vi "APC_9049_CycleAvgSignals.vi"() -> (1 "CRIo9049_CycleAvgSignals":string[](array[string])=["TimeStamp9049_ms", "TimeStamp9056echo_ms", "InjectionState_b", "InjEnable_b", "MainEnable_b", "MainDuration_ms", "MainSOI_CADBTDC", "SparkEnable_b", "SparkTiming_CADBTDC", "EngineSpeed_rpm", "WF-PT-012avg_bar", "WF-PT-005avg_bar", "IMEPg1_bar", "IMEPg2_bar", "IMEPg3_bar", "IMEPg4_bar", "IMEPg5_bar", "IMEPg6_bar", "IMEPn1_bar", "IMEPn2_bar", "IMEPn3_bar", "IMEPn4_bar", "IMEPn5_bar", "IMEPn6_bar", "PMEP1_bar", "PMEP2_bar", "PMEP3_bar", "PMEP4_bar", "PMEP5_bar", "PMEP6_bar", "MaxPcyl1_bar", "MaxPcyl2_bar", "MaxPcyl3_bar", "MaxPcyl4_bar", "MaxPcyl5_bar", "MaxPcyl6_bar", "IMEPstd1_bar", "IMEPstd2_bar", "IMEPstd3_bar", "IMEPstd4_bar", "IMEPstd5_bar", "IMEPstd6_bar", "MAPO1_bar", "MAPO2_bar", "MAPO3_bar", "MAPO4_bar", "MAPO5_bar", "MAPO6_bar", "RI1", "RI2", "RI3", "RI4", "RI5", "RI6", "maxQ1_J", "maxQ2_J", "maxQ3_J", "maxQ4_J", "maxQ5_J", "maxQ6_J", "CA03_1_CADATDC", "CA03_2_CADATDC", "CA03_3_CADATDC", "CA03_4_CADATDC", "CA03_5_CADATDC", "CA03_6_CADATDC", "CA10_1_CADATDC", "CA10_2_CADATDC", "CA10_3_CADATDC", "CA10_4_CADATDC", "CA10_5_CADATDC", "CA10_6_CADATDC", "CA50_1_CADATDC", "CA50_2_CADATDC", "CA50_3_CADATDC", "CA50_4_CADATDC", "CA50_5_CADATDC", "CA50_6_CADATDC", "CA90_1_CADATDC", "CA90_2_CADATDC", "CA90_3_CADATDC", "CA90_4_CADATDC", "CA90_5_CADATDC", "CA90_6_CADATDC", "CA97_1_CADATDC", "CA97_2_CADATDC", "CA97_3_CADATDC", "CA97_4_CADATDC", "CA97_5_CADATDC", "CA97_6_CADATDC", "CA10CA90_1_CAD", "CA10CA90_2_CAD", "CA10CA90_3_CAD", "CA10CA90_4_CAD", "CA10CA90_5_CAD", "CA10CA90_6_CAD", "maxdpdcad1_barCAD", "maxdpdcad2_barCAD", "maxdpdcad3_barCAD", "maxdpdcad4_barCAD", "maxdpdcad5_barCAD", "maxdpdcad6_barCAD", "kappa_comp1_r", "kappa_comp2_r", "kappa_comp3_r", "kappa_comp4_r", "kappa_comp5_r", "kappa_comp6_r", "kappa_exp1_r", "kappa_exp2_r", "kappa_exp3_r", "kappa_exp4_r", "kappa_exp5_r", "kappa_exp6_r", "CylPresWarnings_u64", "CylPresErrors_u64"])   [LabVIEW 2020]
panel:
  in  "CycleRaster":string[](array[string])=["WF-PT-012avg_bar", "WF-PT-005avg_bar", "PrechamberPeakPdiff_bar", "IMEPg1_bar", "IMEPg2_bar", "IMEPg3_bar", "IMEPg4_bar", "IMEPg5_bar", "IMEPg6_bar", "IMEPn1_bar", "IMEPn2_bar", "IMEPn3_bar", "IMEPn4_bar", "IMEPn5_bar", "IMEPn6_bar", "PMEP1_bar", "PMEP2_bar", "PMEP3_bar", "PMEP4_bar", "PMEP5_bar", "PMEP6_bar", "MaxPcyl1_bar", "MaxPcyl2_bar", "MaxPcyl3_bar", "MaxPcyl4_bar", "MaxPcyl5_bar", "MaxPcyl6_bar", "IMEPstd1_bar", "IMEPstd2_bar", "IMEPstd3_bar", "IMEPstd4_bar", "IMEPstd5_bar", "IMEPstd6_bar", "MAPO1_bar", "MAPO2_bar", "MAPO3_bar", "MAPO4_bar", "MAPO5_bar", "MAPO6_bar", "RI1", "RI2", "RI3", "RI4", "RI5", "RI6", "maxQ1_J", "maxQ2_J", "maxQ3_J", "maxQ4_J", "maxQ5_J", "maxQ6_J", "CA03_1_CADATDC", "CA03_2_CADATDC", "CA03_3_CADATDC", "CA03_4_CADATDC", "CA03_5_CADATDC", "CA03_6_CADATDC", "CA10_1_CADATDC", "CA10_2_CADATDC", "CA10_3_CADATDC", "CA10_4_CADATDC", "CA10_5_CADATDC", "CA10_6_CADATDC", "CA50_1_CADATDC", "CA50_2_CADATDC", "CA50_3_CADATDC", "CA50_4_CADATDC", "CA50_5_CADATDC", "CA50_6_CADATDC", "CA90_1_CADATDC", "CA90_2_CADATDC", "CA90_3_CADATDC", "CA90_4_CADATDC", "CA90_5_CADATDC", "CA90_6_CADATDC", "CA97_1_CADATDC", "CA97_2_CADATDC", "CA97_3_CADATDC", "CA97_4_CADATDC", "CA97_5_CADATDC", "CA97_6_CADATDC", "CA10CA90_1_CAD", "CA10CA90_2_CAD", "CA10CA90_3_CAD", "CA10CA90_4_CAD", "CA10CA90_5_CAD", "CA10CA90_6_CAD", "maxdpdcad1_barCAD", "maxdpdcad2_barCAD", "maxdpdcad3_barCAD", "maxdpdcad4_barCAD", "maxdpdcad5_barCAD", "maxdpdcad6_barCAD", "kappa_comp1_r", "kappa_comp2_r", "kappa_comp3_r", "kappa_comp4_r", "kappa_comp5_r", "kappa_comp6_r", "kappa_exp1_r", "kappa_exp2_r", "kappa_exp3_r", "kappa_exp4_r", "kappa_exp5_r", "kappa_exp6_r", "CylPresWarnings_u64", "CylPresErrors_u64"]
  in  "ControlSettingsRaster":string[](array[string])=["InjectionState_b", "InjEnable_b", "MainEnable_b", "MainDuration_ms", "MainSOI_CADBTDC", "SparkEnable_b", "SparkTiming_CADBTDC", "EngineSpeed_rpm"]
  in  "TimeStamp":string[](array[string])=["TimeStamp9049_ms", "TimeStamp9056echo_ms"]
  # "NAMING: for calculated variables, include units on variable names.\n\n_bar \n_degC      (ºC)\n_perc       (%)\n_rpm\n_r              (ratio)\n_b             (bool)\n_u64"
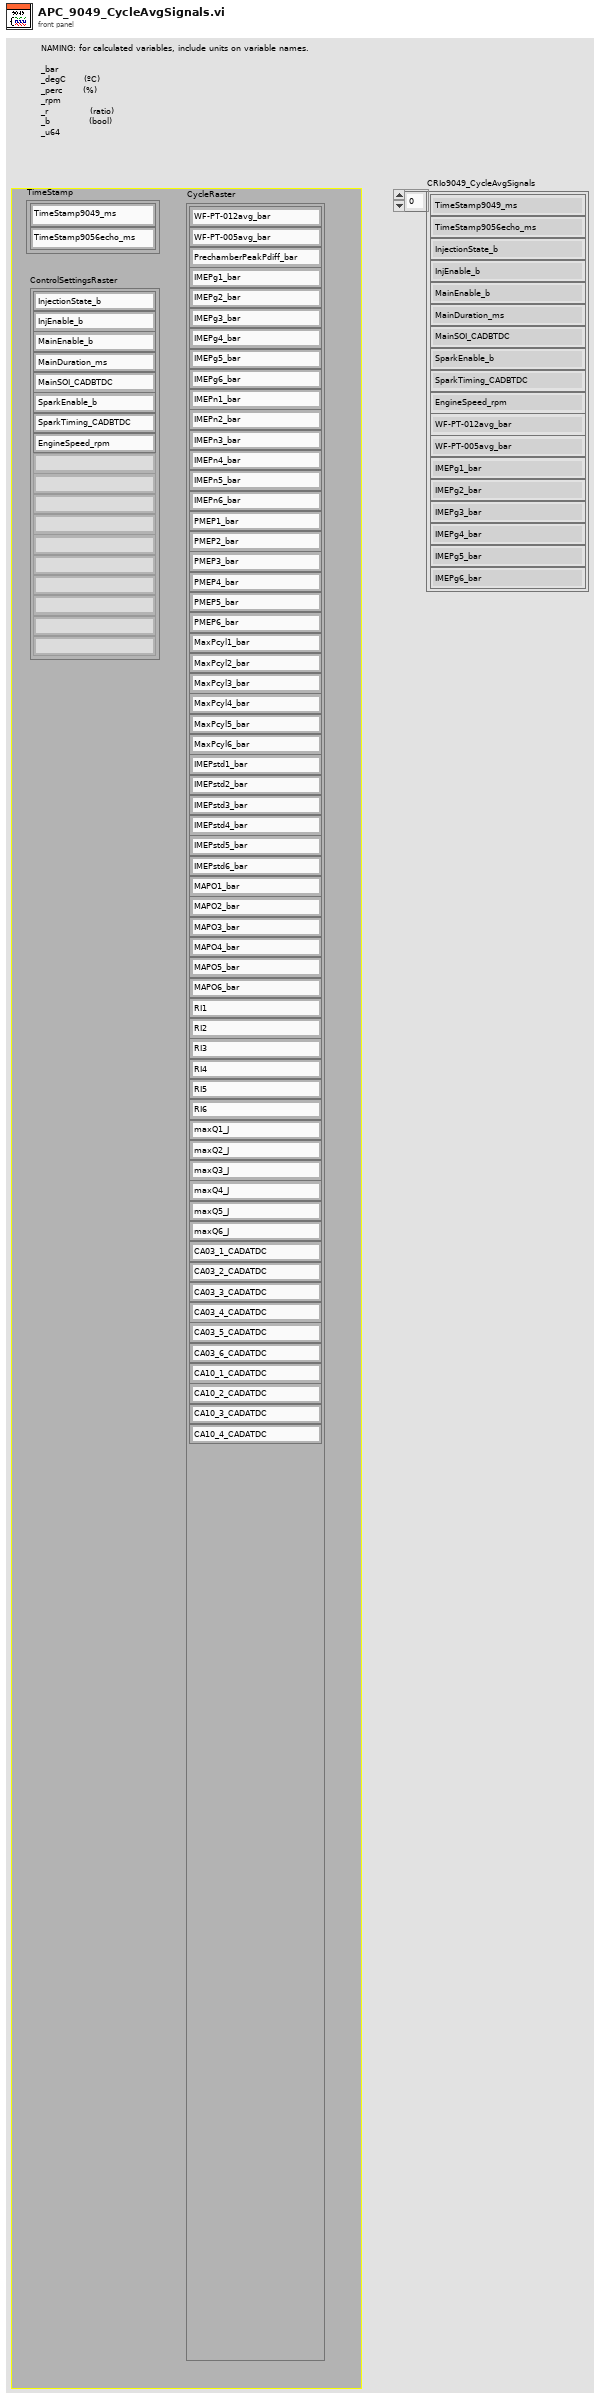
[diagram p1: front panel]
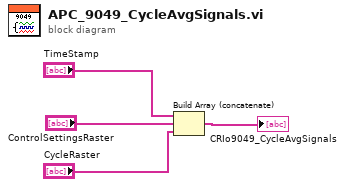
[diagram p0: block diagram]
diagram:
  n1 = Build Array (concatenate)("TimeStamp", "ControlSettingsRaster", "CycleRaster") -> (→"CRIo9049_CycleAvgSignals":string[])
